vi "sub vi - HysteresisCorrectionMatlab (Multiple).vi"(9 "frequency":dbl, 10 "Axis":u16(ring) items=["X", "Y", "Z"], 11 "desired positions":dbl[](array[numeric])) -> (1 "Strain2um":dbl, 3 "correctV":dbl[](array[numeric]))   [LabVIEW 2010]
panel:
  out "Waveform Graph 2":dbl[](graph)
  out "Waveform Graph":dbl[](graph)
  # "About this Program:\n     - Outputs the correct Voltage output neccessary to\n        move the Piezo stage to the desired position"
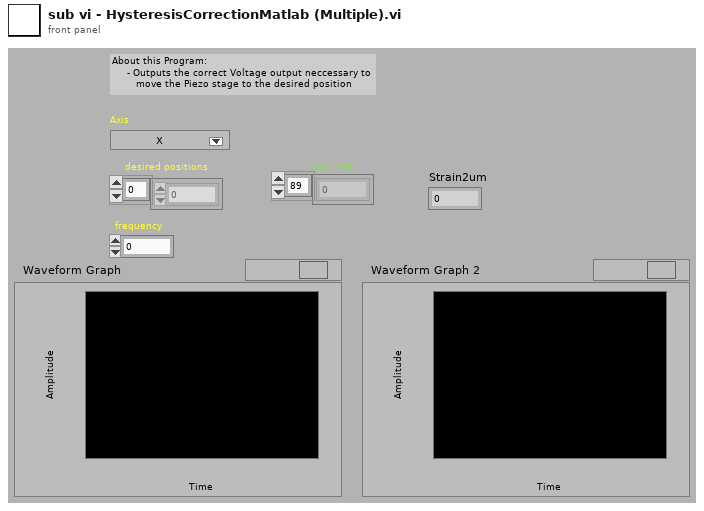
[diagram p1: front panel]
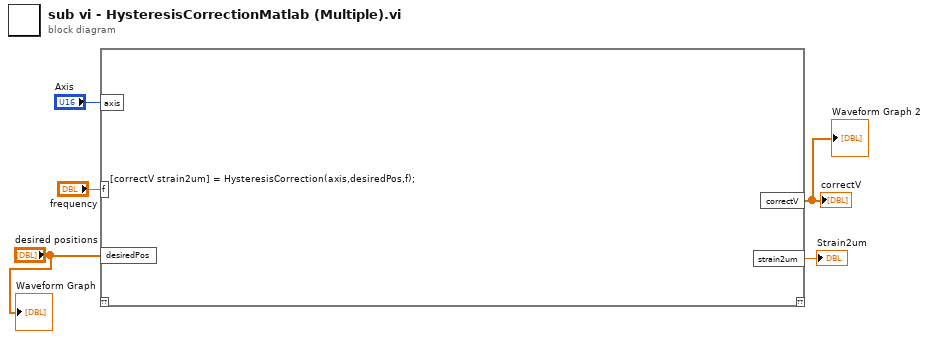
[diagram p0: block diagram]
diagram:
  n1 = script code="[correctV strain2um] = HysteresisCorrection(axis,desiredPos,f);"("desiredPos"="desired positions", "axis"="Axis", "f"="frequency") -> ("correctV"=→"correctV" →"Waveform Graph 2":dbl[], "strain2um"=→"Strain2um":dbl)  [unwired: 2 out]
  "Waveform Graph" <- "desired positions"
